vi "RP100.Measure Current.vi"(8 "error in (no error)":errorcluster, 10 "Output Channel":T1, 11 "VISA resource name":refnum<visa-resource-name>) -> (0 "error out":errorcluster, 1 "measured I":dbl, 2 "Output Channel":T1, 3 "VISA Refnum out":refnum<visa-resource-name>)   [LabVIEW 2016, in "RP100.lvclass"]
uses:
  RP100.lvclass
  Typedefs/Output Channel--Enum.ctl
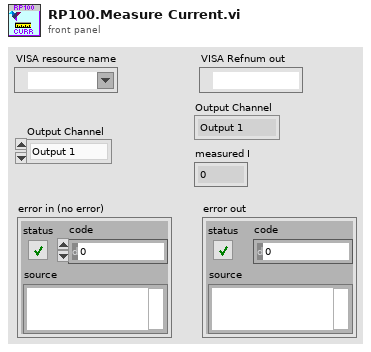
[diagram p1: front panel]
types:
  T1 = typedef "RP100.lvclass/Output Channel--Enum.ctl" = enum16{"Output 1", "Output 2"}
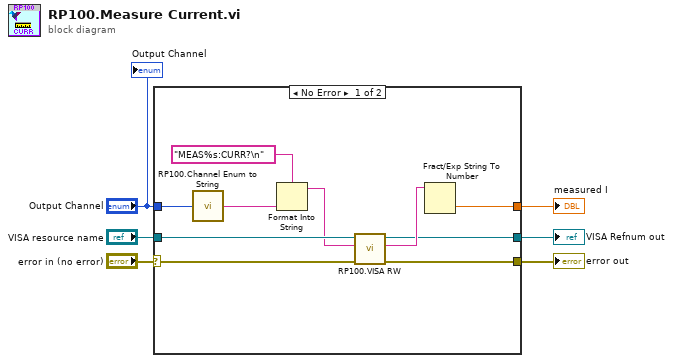
[diagram p0: block diagram]
diagram:
  n1 = case shown="No Error" "error in (no error)" {
    selector: "error in (no error)" -> [w10 w18]
    tunnel: [w7 w17] -> w6
    tunnel: "VISA resource name" -> [w12 w17]
    tunnel: [w9 w18] -> w4
    tunnel: [w16 _] -> w3
    tunnel: "Output Channel" -> [w15 _]
    frame No Error {
      n2 = call "RP100.Channel Enum to String.vi"("OutputChannel"=w15) -> ("format string"=w14:string)
      n3 = Format Into String(format string="MEAS%s:CURR?\n", w14) -> (resulting string=w11:string)  [unwired: 2 in, 1 out]
      n4 = call "RP100.VISA RW.vi"("error in (no error)"=w10, "Write"=w11, "VISA Refnum in"=w12) -> ("error out"=w9:errorcluster, "Read"=w8:string, "VISA Refnum out"=w7:refnum<visa-resource-name>)  [unwired: 6 in]
      n5 = Fract/Exp String To Number(string=w8) -> (number=w16:dbl)  [unwired: 3 in, 1 out]
    }
    frame Error {
    }
  }
  "measured I" <- w3
  "VISA Refnum out" <- w6
  "error out" <- w4
  "Output Channel" <- "Output Channel"
